vi "DROPBEAR_Model_Updating_Postprocessing.vi"(8 "error in (no error)":errorcluster, 11 "DROPBEAR_Model_Updating in":refnum<class "DROPBEAR_Model_Updating.lvclass">) -> (0 "Cycle time":dbl, 1 "Nodal":dynamicdata(graph), 2 "Meter":dynamicdata(graph), 3 "Frequency":dynamicdata(graph))   [LabVIEW 2021, in "DROPBEAR_Model_Updating.lvclass"]
uses:
  DROPBEAR_Model_Updating.lvclass
  DROPBEAR_Model_Updating.lvclass/DROPBEAR_Model_Updating.ctl
  Data_Array/Data_Array.lvclass
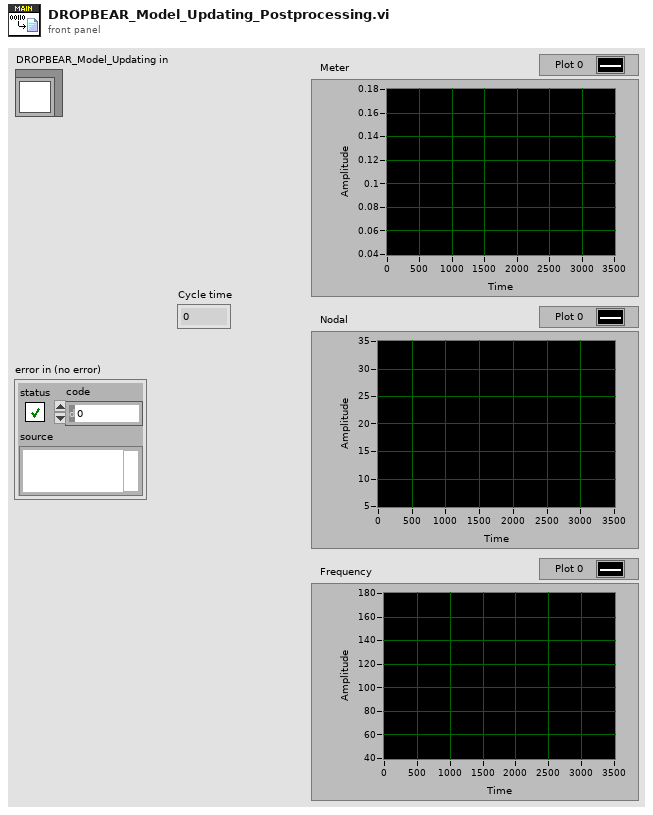
[diagram p1: front panel]
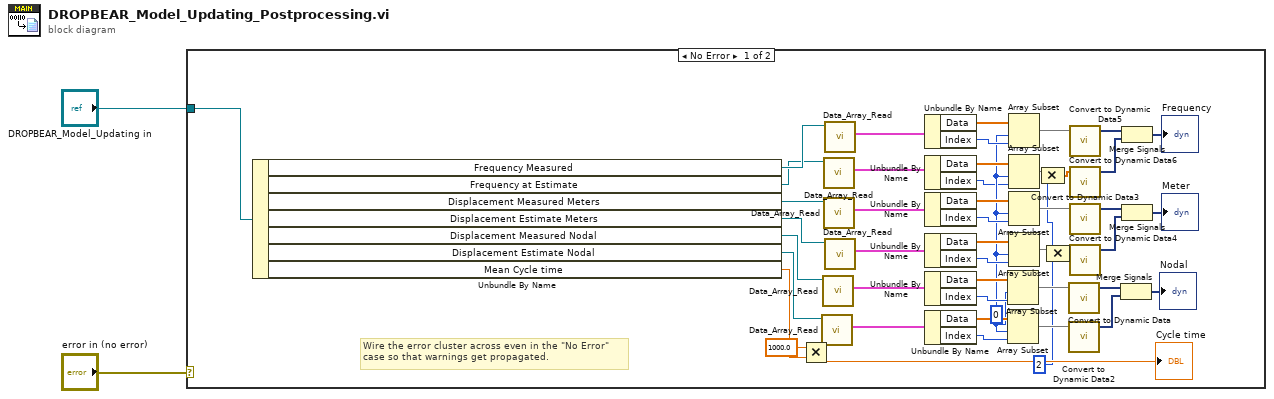
[diagram p0: block diagram]
diagram:
  n1 = case shown="No Error" "error in (no error)" {
    tunnel: "DROPBEAR_Model_Updating in" -> [w49 _]
    frame No Error {
      w3 = 2
      w11 = 0 ("index")
      # "Wire the error cluster across even in the \"No Error\"\ncase so that warnings get propagated."
      n2 = Unbundle By Name(w49) -> ("Frequency Measured"=w10:refnum<class "Data_Array.lvclass">, "Frequency at Estimate"=w9:refnum<class "Data_Array.lvclass">, "Displacement Measured Meters"=w26:refnum<class "Data_Array.lvclass">, "Displacement Estimate Meters"=w27:refnum<class "Data_Array.lvclass">, "Displacement Measured Nodal"=w48:refnum<class "Data_Array.lvclass">, "Displacement Estimate Nodal"=w47:refnum<class "Data_Array.lvclass">, "Mean Cycle time"=w46:dbl)
      n3 = Multiply(x=1000.0, y=w46) -> (x*y=→"Cycle time":dbl)
      n4 = call-dynamic "Data_Array_Read.vi"("Data_Array in"=w47) -> ("Data_params"=w37:cluster{"Data":dbl[], "Index":i32, "Buffer":i32})  [unwired: 8 in, 2 out]
      n5 = call-dynamic "Data_Array_Read.vi"("Data_Array in"=w48) -> ("Data_params"=w36:cluster{"Data":dbl[], "Index":i32, "Buffer":i32})  [unwired: 8 in, 2 out]
      n6 = call-dynamic "Data_Array_Read.vi"("Data_Array in"=w9) -> ("Data_params"=w8:cluster{"Data":dbl[], "Index":i32, "Buffer":i32})  [unwired: 8 in, 2 out]
      n7 = call-dynamic "Data_Array_Read.vi"("Data_Array in"=w26) -> ("Data_params"=w25:cluster{"Data":dbl[], "Index":i32, "Buffer":i32})  [unwired: 8 in, 2 out]
      n8 = call-dynamic "Data_Array_Read.vi"("Data_Array in"=w10) -> ("Data_params"=w7:cluster{"Data":dbl[], "Index":i32, "Buffer":i32})  [unwired: 8 in, 2 out]
      n9 = call-dynamic "Data_Array_Read.vi"("Data_Array in"=w27) -> ("Data_params"=w24:cluster{"Data":dbl[], "Index":i32, "Buffer":i32})  [unwired: 8 in, 2 out]
      n10 = Unbundle By Name(w7) -> ("Data"=w15:dbl[], "Index"=w17:i32)
      n11 = Unbundle By Name(w8) -> ("Data"=w14:dbl[], "Index"=w6:i32)
      n12 = Unbundle By Name(w25) -> ("Data"=w30:dbl[], "Index"=w33:i32)
      n13 = Unbundle By Name(w24) -> ("Data"=w29:dbl[], "Index"=w32:i32)
      n14 = Unbundle By Name(w36) -> ("Data"=w40:dbl[], "Index"=w43:i32)
      n15 = Unbundle By Name(w37) -> ("Data"=w39:dbl[], "Index"=w42:i32)
      n16 = Array Subset(array=w40, index=w11, length=w43) -> (w41:dbl[])
      n17 = Array Subset(array=w39, index=w11, length=w42) -> (w38:dbl[])
      n18 = Array Subset(array=w15, index=w11, length=w17) -> (w16:dbl[])
      n19 = Array Subset(array=w14, index=w11, length=w6) -> (w13:dbl[])
      n20 = Array Subset(array=w30, index=w11, length=w33) -> (w31:dbl[])
      n21 = Array Subset(array=w29, index=w11, length=w32) -> (w28:dbl[])
      n22 = Compound Arithmetic op=MULTIPLY(w13, w3) -> (w4:dbl[])
      n23 = Compound Arithmetic op=MULTIPLY(w28, w3) -> (w5:dbl[])
      n24 = call "Convert to Dynamic Data"("Array"=w41) -> ("Dynamic Data Type"=w45:dynamicdata)  [unwired: 3 in]
      n25 = call "Convert to Dynamic Data2"("Array"=w38) -> ("Dynamic Data Type"=w44:dynamicdata)  [unwired: 3 in]
      n26 = call "Convert to Dynamic Data5"("Array"=w16) -> ("Dynamic Data Type"=w19:dynamicdata)  [unwired: 3 in]
      n27 = call "Convert to Dynamic Data6"("Array"=w4) -> ("Dynamic Data Type"=w18:dynamicdata)  [unwired: 3 in]
      n28 = call "Convert to Dynamic Data3"("Array"=w31) -> ("Dynamic Data Type"=w35:dynamicdata)  [unwired: 3 in]
      n29 = call "Convert to Dynamic Data4"("Array"=w5) -> ("Dynamic Data Type"=w34:dynamicdata)  [unwired: 3 in]
      n30 = Merge Signals(w45, w44) -> (→"Nodal":dynamicdata)
      n31 = Merge Signals(w19, w18) -> (→"Frequency":dynamicdata)
      n32 = Merge Signals(w35, w34) -> (→"Meter":dynamicdata)
    }
    frame Error {
    }
  }
